vi "ReadDBFloat.vi"(2 "start":i32, 3 "db":i32, 4 "PLC":refnum<vi>) -> (0 "value":sgl, 1 "ok":bool)   [LabVIEW 2023]
uses:
  S7Plc.ctl
  D:/Projects/S7View/S7Lib/bin/Debug/S7.Net.dll
  S7Lib/bin/Debug/S7.Net.dll
  D:/Projects/S7View/S7Lib/bin/Debug/S7Lib.dll
  S7Lib/bin/Debug/S7Lib.dll
panel:
  out "错误输出":errorcluster
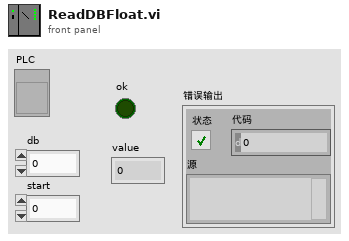
[diagram p1: front panel]
types:
  T1 = typedef "S7Plc.ctl" = cluster{"ip":string, "type":i16, "rack":i16, "slot":i16, "status":bool, "link":bool, "msg":string, "plc":refnum<k24>}
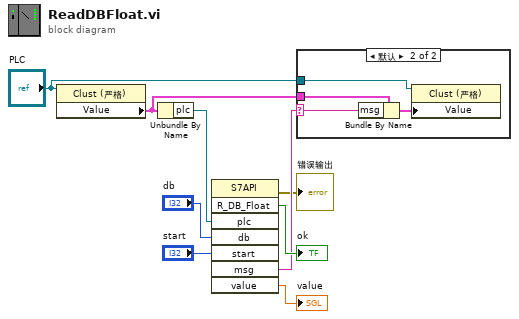
[diagram p0: block diagram]
diagram:
  n1 = property on="属性节点" class="Clust (严格)"(reference="PLC") -> ("Value"=w9:T1)  [unwired: 1 in, 2 out]
  n2 = Unbundle By Name(w9) -> ("plc"=w7:refnum<k24>)
  n3 = invoke on="调用节点" class="S7API" method="R_DB_Float"("plc"=w7, "db"="db", "start"="start") -> (error out=→"错误输出":errorcluster, "R_DB_Float"=→"ok":bool, "msg"=w2:string, "value"=→"value":sgl)  [unwired: 5 in, 4 out]
  n4 = case shown="默认" w2 {
    selector: w2 -> [_ w10]
    tunnel: w9 -> [_ w13]
    tunnel: "PLC" -> [_ w11]
    frame "" {
    }
    frame Default {
      n5 = Bundle By Name(cluster=w13, "msg"=w10) -> (w12:T1)
      n6 = property on="属性节点" class="Clust (严格)"(reference=w11, "Value"=w12) -> ()  [unwired: 1 in, 2 out]
    }
  }
